vi "Main.vi"() -> ()   [LabVIEW 2018]
uses:
  <vilib>/httpClient/LabVIEWHTTPClient.lvlib
panel:
  out "error out":errorcluster
  out "body":string
  out "headers":string
  in  "Tree":string(tree)
  in  "stop":bool
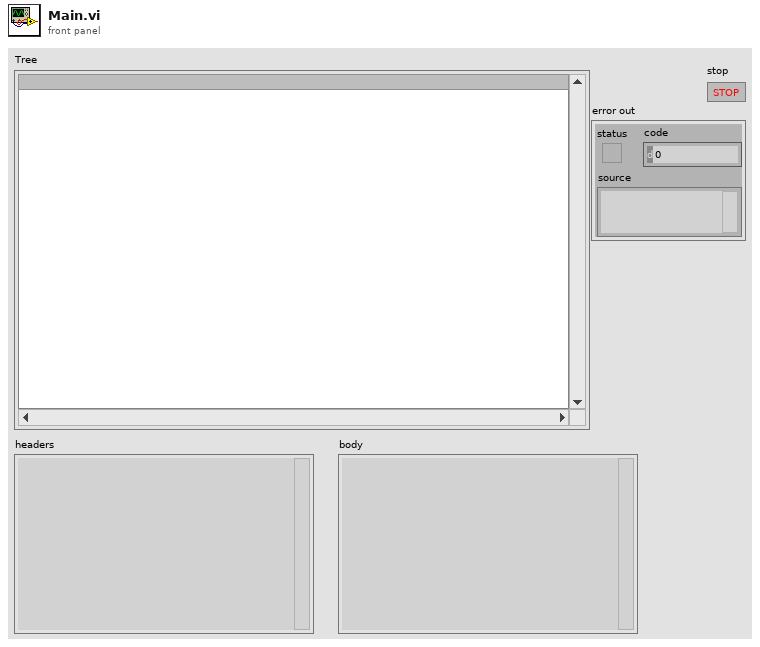
[diagram p1: front panel]
types:
  T1 = typedef "LabVIEWHTTPClient.lvlib/ClientHandle.ctl" = refnum<k1>
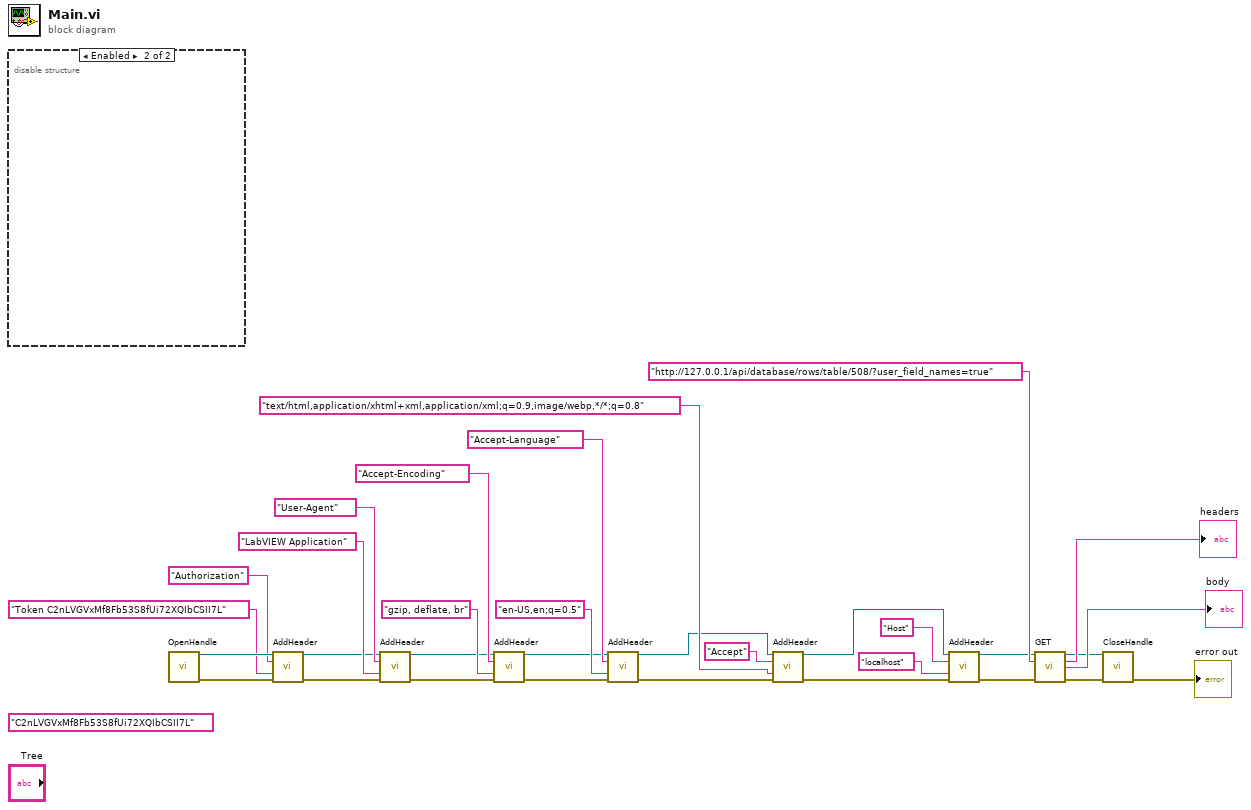
[diagram p0: block diagram]
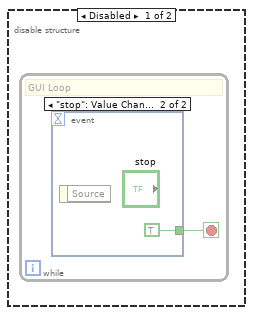
[diagram p2: hidden frame]
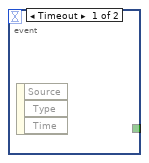
[diagram p3: hidden frame]
diagram:
  (unwired) "C2nLVGVxMf8Fb53S8fUi72XQIbCSII7L" ("secret id")
  n1 = disable-structure shown="Enabled" {
    frame Disabled {
      n2 = while {
        stop <- w33 stop-if-true
        # "GUI Loop"
        n3 = event shown="[1] \"stop\": Value Change" {
          selector: _ -> [_ _]
          dyn-events: _ -> [_ _]
          timeout: _ -> [_ _]
          tunnel: [_ TRUE] -> w33
          event Timeout {
            n4 = event-data() -> ()  [unwired: 1 in, 3 out]
          }
          event "stop": Value Change {
            n5 = event-data() -> ()  [unwired: 1 in, 1 out]
          }
        }
      }
    }
    frame Enabled {
    }
  }
  n6 = call <vilib>:"OpenHandle.vi"() -> ("client handle out"=w27:T1, "error out"=w26:errorcluster)  [unwired: 14 in]
  n7 = call <vilib>:"AddHeader.vi"("client handle"=w27, "header"="Authorization", "value"="Token C2nLVGVxMf8Fb53S8fUi72XQIbCSII7L", "error in (no error)"=w26) -> ("client handle out"=w21:T1, "error out"=w20:errorcluster)  [unwired: 10 in]
  n8 = call <vilib>:"AddHeader.vi"("client handle"=w21, "header"="User-Agent", "value"="LabVIEW Application", "error in (no error)"=w20) -> ("client handle out"=w10:T1, "error out"=w9:errorcluster)  [unwired: 10 in]
  n9 = call <vilib>:"AddHeader.vi"("client handle"=w10, "header"="Accept-Encoding", "value"="gzip, deflate, br", "error in (no error)"=w9) -> ("client handle out"=w12:T1, "error out"=w8:errorcluster)  [unwired: 10 in]
  n10 = call <vilib>:"AddHeader.vi"("client handle"=w12, "header"="Accept-Language", "value"="en-US,en;q=0.5", "error in (no error)"=w8) -> ("client handle out"=w11:T1, "error out"=w7:errorcluster)  [unwired: 10 in]
  n11 = call <vilib>:"AddHeader.vi"("client handle"=w11, "header"="Accept" ("value"), "value"="text/html,application/xhtml+xml,application/xml;q=0.9,image/webp,*/*;q=0.8", "error in (no error)"=w7) -> ("client handle out"=w4:T1, "error out"=w2:errorcluster)  [unwired: 10 in]
  n12 = call <vilib>:"AddHeader.vi"("client handle"=w4, "header"="Host" ("value"), "value"="localhost", "error in (no error)"=w2) -> ("client handle out"=w3:T1, "error out"=w1:errorcluster)  [unwired: 10 in]
  n13 = call <vilib>:"GET.vi"("client handle"=w3, "url"="http://127.0.0.1/api/database/rows/table/508/?user_field_names=true", "error in (no error)"=w1) -> ("client handle out"=w30:T1, "headers"=→"headers":string, "body"=→"body":string, "error out"=w29:errorcluster)  [unwired: 9 in]
  n14 = call <vilib>:"CloseHandle.vi"("client handle"=w30, "error in (no error)"=w29) -> ("error out"=→"error out":errorcluster)  [unwired: 13 in]
